vi "ServoController_setPWM.vi"(0 "Servo Controller Index":u8, 5 "PWM Channel":u8, 7 "On (0)":u16, 9 "Off (duty-cycle)":u16, 11 "Error In":errorcluster) -> (15 "Error Out":errorcluster)   [LabVIEW 2013]
uses:
  <vilib>/myRIO/Instrument Drivers/Onboard IO/I2C/vis/Smart Open.vi
  <vilib>/myRIO/Instrument Drivers/Onboard IO/I2C/vis/Configure.vi
  <vilib>/myRIO/Instrument Drivers/Onboard IO/I2C/vis/Write.vi
  <vilib>/myRIO/Instrument Drivers/Onboard IO/I2C/vis/Open.vi
  <vilib>/myRIO/Common/Instrument Driver Framework/myRIO v1.0/I2C/vis/myRIO v1.1 Open I2C.vi
  <vilib>/myRIO/Common/Instrument Driver Framework/Utilities/vis/Validate Channels.vi
  <vilib>/myRIO/Common/Instrument Driver Framework/myRIO v1.0/I2C/vis/myRIO v1.0 Reserve I2C.vi
  <vilib>/myRIO/Common/Instrument Driver Framework/myRIO v1.0/I2C/vis/myRIO v1.0 Build MUX Configuration I2C.vi
  <vilib>/myRIO/Common/Instrument Driver Framework/myRIO v1.0/Resource Manager/vis/myRIO v1.0 Reserve Channel List.vi
  <vilib>/myRIO/Common/Instrument Driver Framework/myRIO v1.0/Resource Manager/vis/myRIO v1.0 Create Configuration List.vi
  <vilib>/myRIO/Common/Instrument Driver Framework/myRIO v1.0/Resource Manager/vis/myRIO v1.0 Reserve Channel.vi
  <vilib>/myRIO/Common/Instrument Driver Framework/myRIO v1.0/Resource Manager/vis/myRIO v1.0 Unreserve Channel.vi
  <vilib>/myRIO/Common/Instrument Driver Framework/myRIO v1.0/Resource Manager/vis/myRIO v1.0 Build Mutex Name.vi
  <vilib>/myRIO/Common/Instrument Driver Framework/myRIO v1.0/myRIO v1.1 Open.vi
  <vilib>/Utility/VariantDataType/GetNumericInfo.vi
  <vilib>/Utility/error.llb/Error Cluster From Error Code.vi
  <vilib>/myRIO/Common/Instrument Driver Framework/Utilities/vis/IO Manager.vi
  <vilib>/myRIO/Common/Instrument Driver Framework/Utilities/vis/Configuration Manager.vi
  <vilib>/myRIO/Common/Instrument Driver Framework/myRIO v1.0/Resource Manager/vis/myRIO v1.0 Configure IO.vi
  <vilib>/myRIO/Common/Instrument Driver Framework/myRIO v1.0/myRIO v1.0 Close.vi
  <vilib>/myRIO/Common/Instrument Driver Framework/myRIO v1.0/I2C/vis/myRIO v1.0 Configure I2C.vi
  <vilib>/myRIO/Common/Instrument Driver Framework/myRIO v1.0/I2C/vis/myRIO v1.0 Write I2C.vi
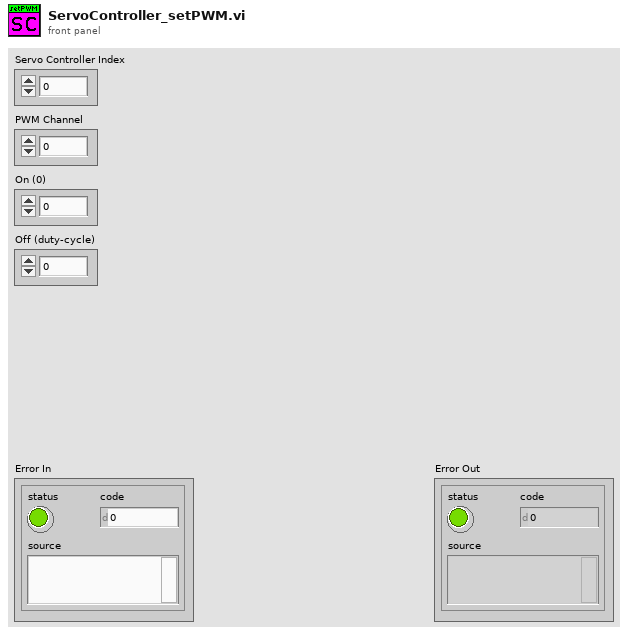
[diagram p1: front panel]
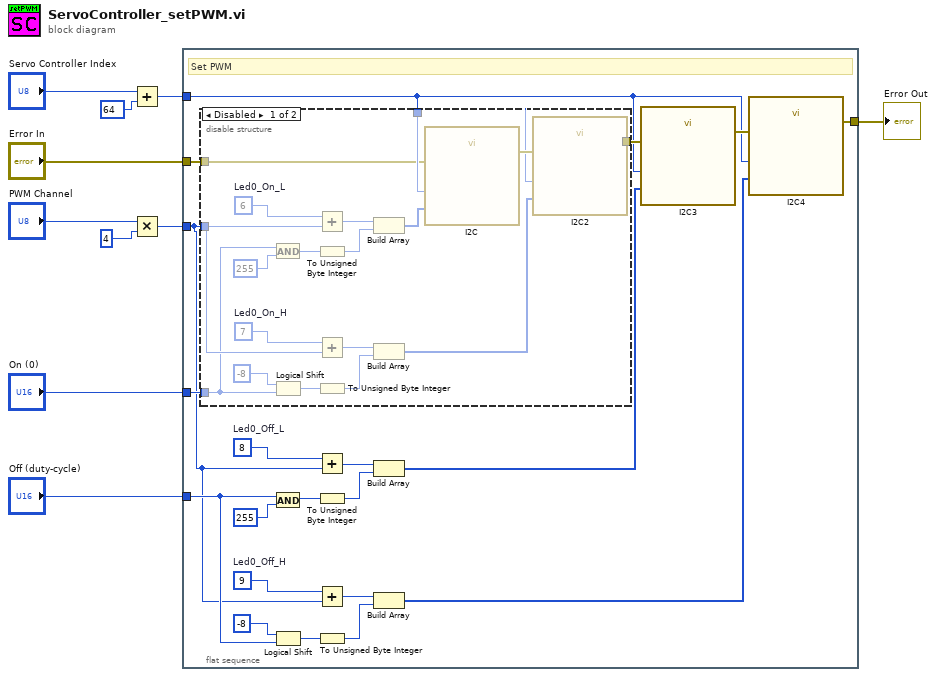
[diagram p0: block diagram]
diagram:
  n1 = Add(x="Servo Controller Index", y=u8 64 ("Slave Address (7-bit)")) -> (x+y=w9:u8)
  n2 = Multiply(x="PWM Channel", y=u8 4) -> (x*y=w7:u8)
  n3 = flat-sequence {
    tunnel: w9 -> [w14]
    tunnel: [w21] -> w2
    tunnel: w7 -> [w11]
    tunnel: "On (0)" -> [w13]
    tunnel: "Off (duty-cycle)" -> [w24]
    tunnel: "Error In" -> [w12]
    frame #0 {
      w29 = u8 9  # Led0_Off_H
      w30 = u8 8  # Led0_Off_L
      # "Set PWM"
      n4 = disable-structure shown="Disabled" {
        disable-tunnel: [w38 w49] -> w23
        disable-tunnel: w14 -> [w34 _]
        disable-tunnel: w11 -> [w33 _]
        disable-tunnel: w13 -> [w32 _]
        disable-tunnel: w12 -> [w31 w49]
        frame Disabled {
          w47 = u8 7  # Led0_On_H
          w48 = u8 6  # Led0_On_L
          n5 = And(x=w32, y=u16 255) -> (x .and. y?=w43:u16)
          n6 = Logical Shift(y=i8 -8 ("x"), x=w32) -> (x << y=w42:u16)
          n7 = Add(x=w48, y=w33) -> (x+y=w46:u8)
          n8 = To Unsigned Byte Integer(number=w43) -> (unsigned 8bit integer=w44:u8)
          n9 = Add(x=w47, y=w33) -> (x+y=w37:u8)
          n10 = To Unsigned Byte Integer(number=w42) -> (unsigned 8bit integer=w36:u8)
          n11 = Build Array(w46, w44) -> (w40:u8[])
          n12 = Build Array(w37, w36) -> (w35:u8[])
          n13 = call "I2C"("Slave Address (7-bit)"=w34, "Bytes to Write"=w40, "error in (no error)"=w31) -> ("error out"=w39:errorcluster)  [unwired: 24 in]
          n14 = call "I2C2"("Slave Address (7-bit)"=w34, "Bytes to Write"=w35, "error in (no error)"=w39) -> ("error out"=w38:errorcluster)  [unwired: 24 in]
        }
        frame Enabled {
        }
      }
      n15 = And(x=w24, y=u16 255) -> (x .and. y?=w28:u16)
      n16 = Logical Shift(y=i8 -8 ("x"), x=w24) -> (x << y=w25:u16)
      n17 = Add(x=w30, y=w11) -> (x+y=w19:u8)
      n18 = To Unsigned Byte Integer(number=w28) -> (unsigned 8bit integer=w18:u8)
      n19 = Add(x=w29, y=w11) -> (x+y=w17:u8)
      n20 = To Unsigned Byte Integer(number=w25) -> (unsigned 8bit integer=w16:u8)
      n21 = Build Array(w19, w18) -> (w20:u8[])
      n22 = Build Array(w17, w16) -> (w15:u8[])
      n23 = call "I2C3"("Slave Address (7-bit)"=w14, "Bytes to Write"=w20, "error in (no error)"=w23) -> ("error out"=w22:errorcluster)  [unwired: 24 in]
      n24 = call "I2C4"("Slave Address (7-bit)"=w14, "Bytes to Write"=w15, "error in (no error)"=w22) -> ("error out"=w21:errorcluster)  [unwired: 24 in]
    }
  }
  "Error Out" <- w2
